vi "SearchStringBenchmark.vi"() -> ()   [LabVIEW 2017]
uses:
  SearchStr.dll
panel:
  out "offset of match":i32
  in  "Type":enum16{"AVX2", "AVX512"}(ring)
  out "Time, DLL, s":dbl
  out "Time, LabVIEW, s":dbl
  out "Pass":bool
  out "Ratio":dbl
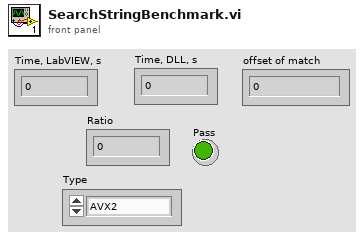
[diagram p1: front panel]
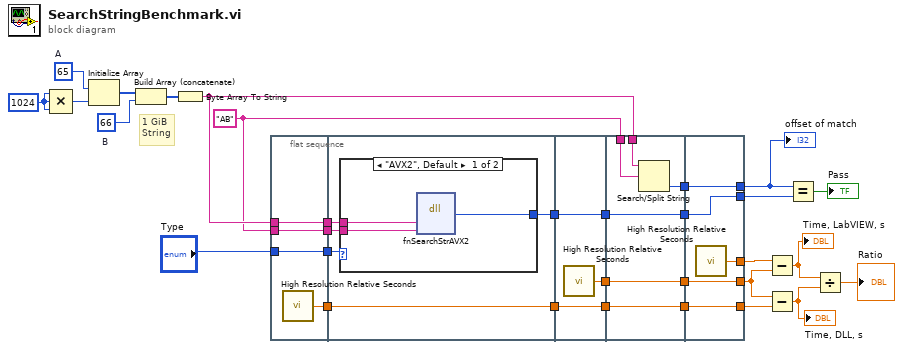
[diagram p0: block diagram]
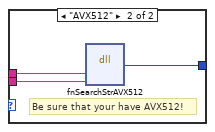
[diagram p2: hidden frame]
diagram:
  w21 = u8 66  # B
  w29 = u8 65  # A
  w30 = 1024
  w3 = "AB"
  # "1 GiB\nString"
  n1 = Compound Arithmetic op=MULTIPLY(w30, w30, w30) -> (w23:i32)
  n2 = Initialize Array(w29, w23) -> (w22:u8[])
  n3 = Build Array (concatenate)(w22, w21) -> (w20:u8[])
  n4 = Byte Array To String(unsigned byte array=w20) -> (string=w13:string)
  n5 = flat-sequence {
    tunnel: w13 -> [w34]
    tunnel: w3 -> [w35]
    tunnel: [w35] -> w28
    tunnel: [w34] -> w27
    tunnel: [w33] -> w26
    tunnel: [w32] -> w2
    tunnel: "Type" -> [w32]
    tunnel: w28 -> [w37]
    tunnel: w27 -> [w40]
    tunnel: w26 -> [w39]
    tunnel: [w39] -> w25
    tunnel: [w38] -> w24
    tunnel: w2 -> [w36]
    tunnel: w25 -> [w48]
    tunnel: w24 -> [w47]
    tunnel: [w49] -> w19
    tunnel: [w48] -> w18
    tunnel: [w47] -> w17
    tunnel: w19 -> [w55]
    tunnel: w18 -> [w54]
    tunnel: w17 -> [w53]
    tunnel: w13 -> [w52]
    tunnel: [w55] -> w16
    tunnel: [w54] -> w15
    tunnel: [w53] -> w14
    tunnel: [w51] -> w12
    tunnel: w3 -> [w50]
    tunnel: [w59] -> w4
    tunnel: [w60] -> w8
    tunnel: w16 -> [w60]
    tunnel: w15 -> [w56]
    tunnel: w14 -> [w59]
    tunnel: [w58] -> w11
    tunnel: w12 -> [w58]
    tunnel: [w57] -> w9
    tunnel: [w56] -> w7
    frame #0 {
      n6 = call <vilib>:"High Resolution Relative Seconds.vi"() -> ("relative seconds"=w33:dbl)
    }
    frame #1 {
      n7 = case shown="\"AVX2\", Default" w36 {
        tunnel: w40 -> [w43 w46]
        tunnel: [w42 w45] -> w38
        tunnel: w37 -> [w41 w44]
        frame "AVX2", Default {
          n8 = dll-call lib="C:/Users/Andrey/Desktop/SlowString&Search/SearchStringBenchmark/SearchStr.dll" fn="fnSearchStrAVX2"("str_in"=w43, "pattern"=w41) -> ("return type"=w42:i32)  [unwired: 5 in, 2 out]
        }
        frame "AVX512" {
          # "Be sure that your have AVX512!"
          n9 = dll-call lib="C:/Users/Andrey/Desktop/SlowString&Search/SearchStringBenchmark/SearchStr.dll" fn="fnSearchStrAVX512"("str_in"=w46, "pattern"=w44) -> ("return type"=w45:i32)  [unwired: 5 in, 2 out]
        }
      }
    }
    frame #2 {
      n10 = call <vilib>:"High Resolution Relative Seconds.vi"() -> ("relative seconds"=w49:dbl)
    }
    frame #3 {
      n11 = Search/Split String(string=w52, search string/char (-)=w50) -> (offset of match=w51:i32)  [unwired: 1 in, 2 out]
    }
    frame #4 {
      n12 = call <vilib>:"High Resolution Relative Seconds.vi"() -> ("relative seconds"=w57:dbl)
    }
  }
  n13 = Subtract(x=w9, y=w8) -> (x-y=w6:dbl)
  "Time, LabVIEW, s" <- w6
  n14 = Subtract(x=w8, y=w7) -> (x-y=w5:dbl)
  "Time, DLL, s" <- w5
  n15 = Equal?(x=w11, y=w4) -> (x = y?=→"Pass":bool)
  n16 = Divide(x=w6, y=w5) -> (x/y=→"Ratio":dbl)
  "offset of match" <- w11
